vi "LoadSyringeConfiguration.vi"(0 "object in":refnum<class "CetoniPump.lvclass">, 2 "configuration file path":path, 5 "error in (no error)":errorcluster) -> (14 "object out":refnum<class "CetoniPump.lvclass">, 16 "All Found":bool, 17 "Read 2":T1(array[cluster]), 19 "error out":errorcluster)   [LabVIEW 2021, in "CetoniPump.lvclass"]
uses:
  CetoniPump.lvclass
  CetoniPump.lvclass/CetoniPump.ctl
  <vilib>/Utility/config.llb/NI_LVConfig.lvlib
  <vilib>/Utility/config.llb/Read Key (Double).vi
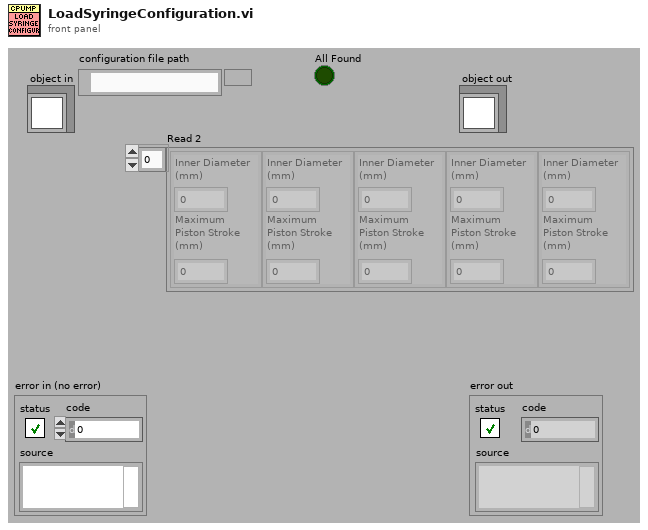
[diagram p1: front panel]
types:
  T1 = cluster{"Inner Diameter \n(mm)":dbl, "Maximum \nPiston Stroke \n(mm)":dbl}[]
  T2 = typedef "NI_LVConfig.lvlib/Config Data RefNum.ctl" = refnum<k1>
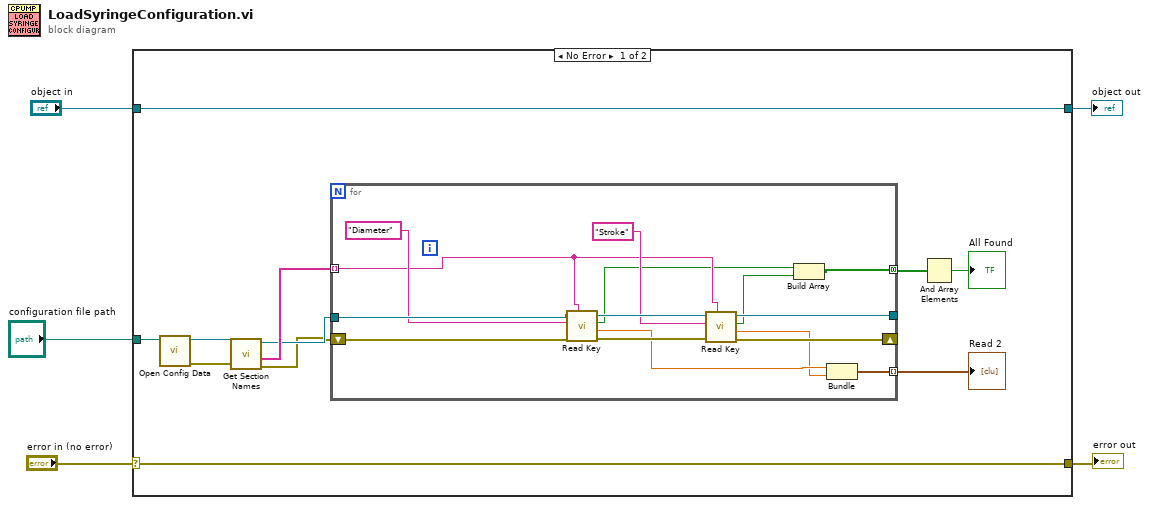
[diagram p0: block diagram]
diagram:
  n1 = case shown="No Error" "error in (no error)" {
    selector: "error in (no error)" -> [w16 w33]
    tunnel: [w16 w33] -> w4
    tunnel: [w15 w32] -> w2
    tunnel: "object in" -> [w15 w32]
    tunnel: "configuration file path" -> [w8 _]
    frame No Error {
      n2 = call <vilib>:"Open Config Data.vi"("configuration file path"=w8) -> ("error out"=w7:errorcluster, "refnum"=w14:T2)  [unwired: 8 in, 1 out]
      n3 = call <vilib>:"Get Section Names.vi"("error in (no error)"=w7, "refnum"=w14) -> ("error out"=w6:errorcluster, "section names"=w13:string[], "refnum out"=w12:T2)  [unwired: 7 in]
      n4 = for {
        tunnel: w12 -> [w31]
        tunnel: [w29] -> _
        shift-right: [w28] -> _
        shift-left: w6 -> [w26]
        tunnel: w13 -> [w20] mode=indexing
        tunnel: [w21] -> w11 mode=indexing
        tunnel: [w17] -> w10 mode=concatenating
        n5 = call-poly <vilib>:"Read Key.vi"("section"=w20, "error in (no error)"=w26, "key"="Diameter", "refnum"=w31) -> ("error out"=w27:errorcluster, "value"=w23:dbl, "found?"=w19:bool, "refnum out"=w30:T2)  [unwired: 4 in]
        n6 = call-poly <vilib>:"Read Key.vi"("section"=w20, "error in (no error)"=w27, "key"="Stroke", "refnum"=w30) -> ("error out"=w28:errorcluster, "value"=w22:dbl, "found?"=w18:bool, "refnum out"=w29:T2)  [unwired: 4 in]
        n7 = Build Array(w19, w18) -> (w17:bool[])
        n8 = Bundle("value"=w23, "value"=w22) -> (w21:cluster{"value":dbl, "value":dbl})  [unwired: 1 in]
      }
      "Read 2" <- w11
      n9 = And Array Elements(Boolean array=w10) -> (logical AND=→"All Found":bool)
    }
    frame Error {
    }
  }
  "error out" <- w4
  "object out" <- w2
